vi "Source Monitor Data.vi"(8 "error in (no error)":errorcluster, 11 "VISA resource name":refnum<visa-resource-name>) -> (0 "error out":errorcluster, 1 "IAC monitor":dbl format="%.4f", 2 "VAC monitor":dbl format="%.4f", 3 "VISA resource name out":refnum<visa-resource-name>)   [LabVIEW 2015, in "Agilent 428X Series.lvlib"]
doc: "The Source Monitor VAC/IAC VI sets the latest measured voltage/current monitor data into the HP 428XA's output buffer."
uses:
  <instrlib>/Agilent 428X Series/Agilent 428X Series.lvlib
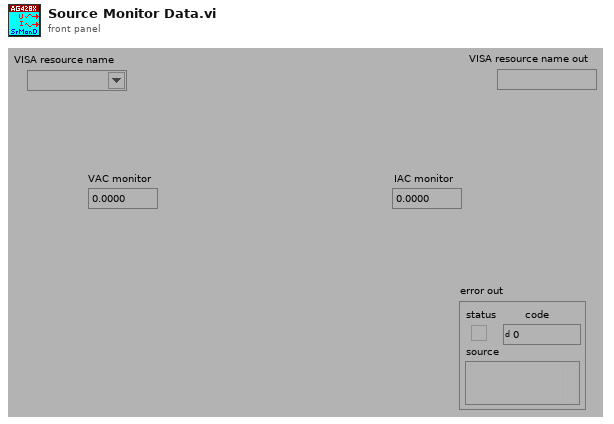
[diagram p1: front panel]
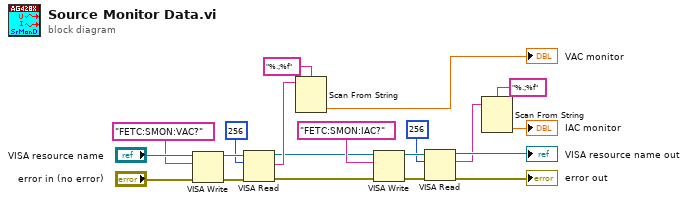
[diagram p0: block diagram]
diagram:
  n1 = VISA Write(VISA resource name="VISA resource name", write buffer="FETC:SMON:VAC?" ("write buffer (\"\")"), error in (no error)="error in (no error)") -> (VISA resource name out=w19:refnum<visa-resource-name>, error out=w17:errorcluster)  [unwired: 1 out]
  n2 = VISA Read(VISA resource name=w19, byte count=u32 256 ("byte count (0)"), error in (no error)=w17) -> (VISA resource name out=w7:refnum<visa-resource-name>, read buffer=w14:string, error out=w4:errorcluster)  [unwired: 1 out]
  n3 = Scan From String(format string="%.;%f", input string=w14) -> (output 1=→"VAC monitor":dbl)  [unwired: 3 in, 3 out]
  n4 = VISA Write(VISA resource name=w7, write buffer="FETC:SMON:IAC?" ("write buffer (\"\")"), error in (no error)=w4) -> (VISA resource name out=w11:refnum<visa-resource-name>, error out=w10:errorcluster)  [unwired: 1 out]
  n5 = VISA Read(VISA resource name=w11, byte count=u32 256 ("byte count (0)"), error in (no error)=w10) -> (VISA resource name out=→"VISA resource name out":refnum<visa-resource-name>, read buffer=w2:string, error out=→"error out":errorcluster)  [unwired: 1 out]
  n6 = Scan From String(format string="%.;%f", input string=w2) -> (output 1=→"IAC monitor":dbl)  [unwired: 3 in, 3 out]
